vi "COMSOL to 1D Array of Waveforms.vi"(7 "COMSOL Data":dbl[][](array[numeric])) -> (8 "1D Array of Waveforms":waveform(dbl)[](array[waveform]))   [LabVIEW 2013]
panel:
  out "Waveform Graph":waveform(dbl)(graph)
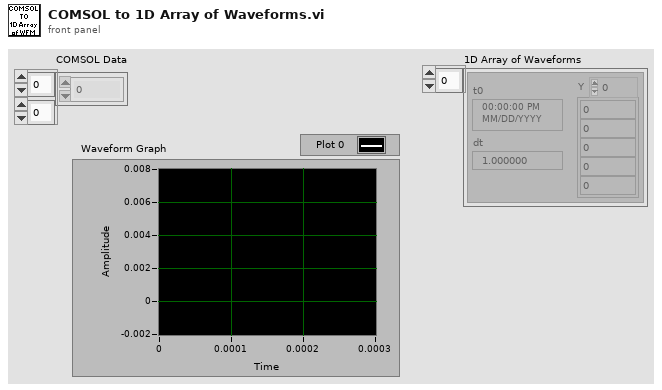
[diagram p1: front panel]
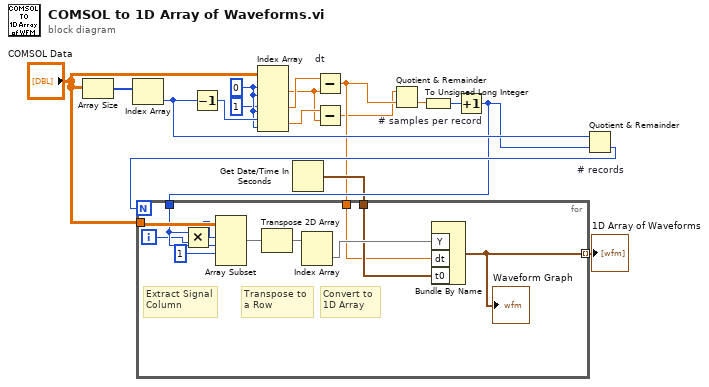
[diagram p0: block diagram]
diagram:
  w12 = 0 ("disabled index (col)")
  n1 = Array Size(array="COMSOL Data") -> (size(s)=w17:i32[])
  n2 = Index Array(array=w17) -> (element=w8:i32)  [unwired: 1 in]
  n3 = Decrement(x=w8) -> (x-1=w16:i32)
  n4 = Index Array(array="COMSOL Data", index (row) #1=w12, index (col) #1=w12, index (row) #2=1 ("disabled index (row)"), index (col) #2=w12, index (row) #3=w16, index (col) #3=w12) -> (element #1=w13:dbl, element #2=w14:dbl, element #3=w15:dbl)
  n5 = Get Date/Time In Seconds() -> (seconds since 1Jan1904=w3:timestamp)
  n6 = Subtract "dt"(x=w14, y=w13) -> (x-y=w2:dbl)
  n7 = Subtract ("difference")(x=w15, y=w13) -> (x-y=w1:dbl)
  n8 = Quotient & Remainder(x=w1, y=w2) -> (floor(x/y)=w10:dbl)  [unwired: 1 out]
  n9 = To Unsigned Long Integer(number=w10) -> (unsigned 32bit integer=w9:u32)
  n10 = Increment "# samples per record"(x=w9) -> (x+1=w5:u32)
  n11 = Quotient & Remainder "# records"(x=w8, y=w5) -> (floor(x/y)=w7:u32)  [unwired: 1 out]
  n12 = for {
    N: w7 -> [_]
    tunnel: "COMSOL Data" -> [w28]
    tunnel: w5 -> [w20]
    tunnel: w2 -> [w18]
    tunnel: [w22] -> w4 mode=indexing
    tunnel: w3 -> [w23]
    i -> [w19]
    # "Convert to\n1D Array"
    # "Transpose to\na Row"
    # "Extract Signal\nColumn"
    n13 = Multiply(x=w20, y=w19) -> (x*y=w21:u32)
    n14 = Array Subset(array=w28, index (row)=w21, length (row)=w20, index (col)=1 ("index")) -> (w26:dbl[][])  [unwired: 1 in]
    n15 = Transpose 2D Array(2D array=w26) -> (transposed array=w25:dbl[][])
    n16 = Index Array(array=w25) -> (element=w24:dbl[])  [unwired: 2 in]
    n17 = Bundle By Name("Y"=w24, "dt"=w18, "t0"=w23) -> (w22:waveform(dbl))  [unwired: 1 in]
    "Waveform Graph" <- w22
  }
  "1D Array of Waveforms" <- w4
